vi "Main Engine Stream Process.vi"(8 "error in (no error)":errorcluster, 10 "Refs":T1, 11 "Process in":refnum<class "Process.lvclass">) -> (0 "error out":errorcluster)   [LabVIEW 2019, in "CAN Streaming Support Engine.lvlib"]
uses:
  CAN Streaming Support Engine.lvlib
  <vilib>/NI/NIVS Inline Async API/_VS Inline Async API/Process/Process.lvclass
  Types/Engine Stream API Refs.ctl
  <vilib>/xnet/xnet.llb/XNET Frame CAN.ctl
  <vilib>/xnet/xnet.llb/XNET Frame Type CAN.ctl
  Types/Engine Stream State.ctl
  <vilib>/NI/NIVS Inline Async API/_VS Inline Async API/Process/Process.lvclass/Process.ctl
  <vilib>/NI/NIVS Inline Async API/_VS Inline Async API/Error Handling Process/SubVIs/Error.ConvertArray.vi
  <vilib>/xnet/xnet.llb/XNET Read (Frame CAN).vi
  <vilib>/Utility/SystemLogging/Write to System Log.vi
  <vilib>/xnet/xnet.llb/XNET Create Session (Frame Input Stream).vi
  <vilib>/ErrorRing/Error Ring.xnode
  <resource>/objmgr/xnet.rc
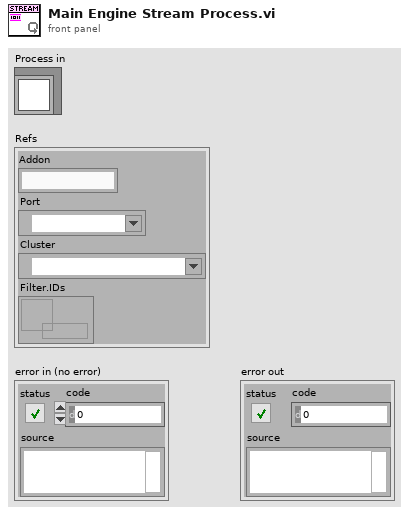
[diagram p1: front panel]
types:
  T1 = typedef "CAN Streaming Support Engine.lvlib/Engine Stream API Refs.ctl" = cluster{"Addon":string, "Port":refnum<k21>, "Cluster":refnum<k21>, "Filter.IDs":refnum<data-value>}
  T2 = typedef "CAN Streaming Support Engine.lvlib/Engine Stream State.ctl" = enum8{"Check for Connection", "Open XNET Session", "Publish", "Cleanup", "Exit"}
  T3 = typedef "XNET Frame CAN.ctl" = cluster{"timestamp":timestamp, "payload":u8[], "identifier":u32, "type":T4, "extended?":bool, "echo?":bool}
  T4 = typedef "XNET Frame Type CAN.ctl" = u8
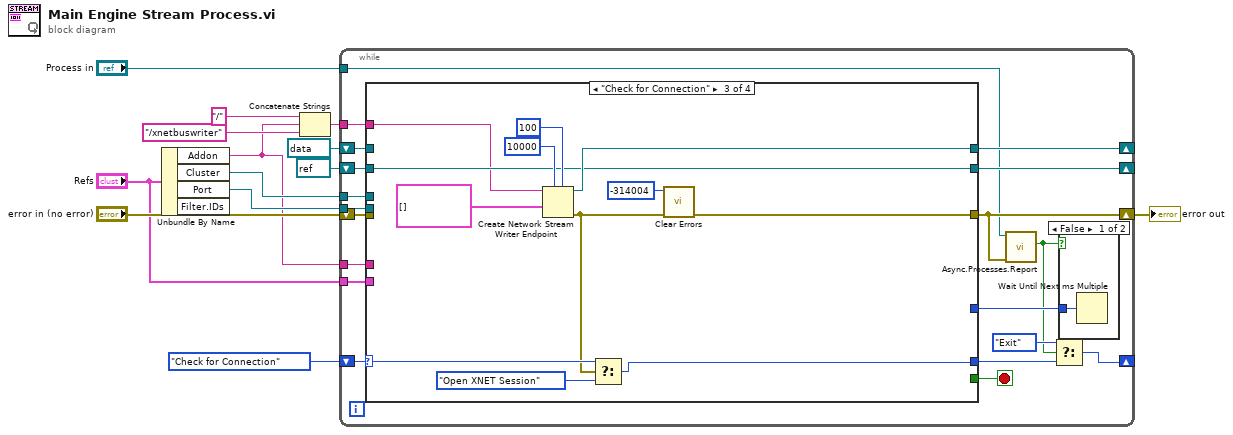
[diagram p0: block diagram]
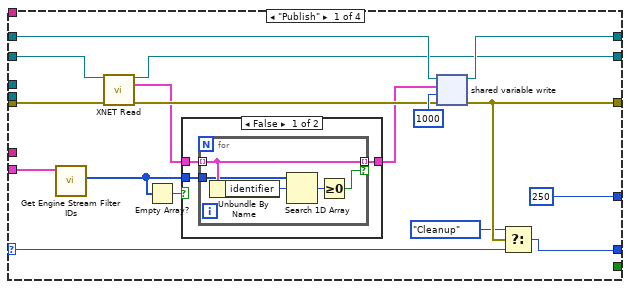
[diagram p2: hidden frame]
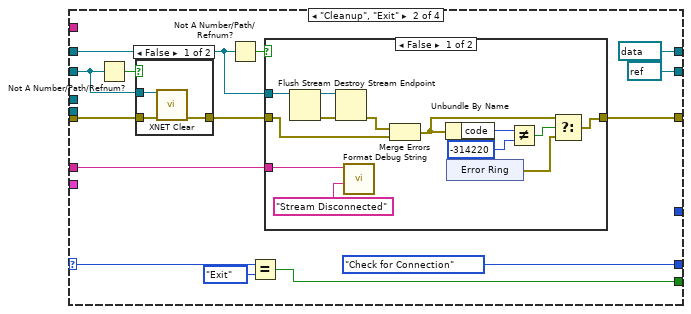
[diagram p4: hidden frame]
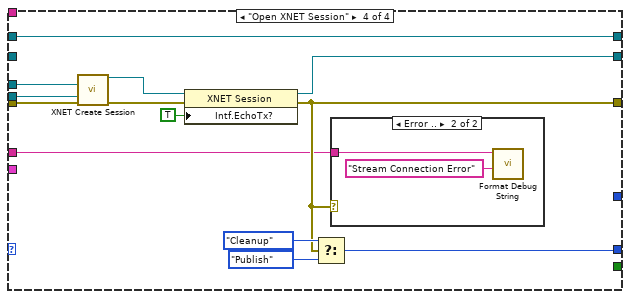
[diagram p7: hidden frame]
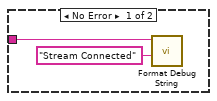
[diagram p8: hidden frame]
diagram:
  n1 = Unbundle By Name("Refs") -> ("Addon"=w1:string, "Cluster"=w13:refnum<k21>, "Port"=w12:refnum<k21>)  [unwired: 1 out]
  n2 = Concatenate Strings("/" ("string"), w1, "/xnetbuswriter" ("reader url")) -> (w8:string)
  n3 = while {
    shift-right: [w18] -> _
    shift-left: Engine_Stream_State."Check for Connection" -> [w32]
    shift-right: [w31] -> _
    shift-left: refnum<k21> refnum ("reader url") -> [w30]
    shift-right: [w21] -> w6
    shift-left: "error in (no error)" -> [w29]
    tunnel: w12 -> [w27]
    shift-right: [w26] -> _
    shift-left: refnum<k21> refnum ("session out") -> [w25]
    tunnel: w8 -> [w23]
    tunnel: w13 -> [w22]
    tunnel: "Process in" -> [w17]
    tunnel: "Refs" -> [w15]
    tunnel: w1 -> [w14]
    stop <- w28 stop-if-true
    n4 = case shown="\"Check for Connection\"" w32 {
      selector: w32 -> [w45 w70 w100 _]
      tunnel: [w44 Engine_Stream_State."Check for Connection" w98 w106] -> w19
      tunnel: [w47 refnum<k21> refnum ("reader url") w97 w107] -> w31
      tunnel: w30 -> [w48 w67 _ w107]
      tunnel: [w46 w60 w93 w105] -> w21
      tunnel: w29 -> [w36 w62 _ w116]
      tunnel: [_ w68 _ _] -> w28
      tunnel: w27 -> [_ _ _ w115]
      tunnel: [w39 refnum<k21> refnum ("session out") w96 w111] -> w26
      tunnel: w25 -> [w42 w64 w96 _]
      tunnel: [u32 250 ("millisecond multiple") _ _ _] -> w24
      tunnel: w23 -> [_ _ w95 _]
      tunnel: w22 -> [_ _ _ w112]
      tunnel: w15 -> [w34 _ _ _]
      tunnel: w14 -> [_ w59 _ w104]
      frame "Publish" {
        n5 = call "Get Engine Stream Filter IDs.vi"("Refs"=w34) -> ("IDs"=w33:u32[])  [unwired: 9 in, 1 out]
        n6 = call-poly <vilib>:"XNET Read.vi"("session in"=w42, "error in (no error)"=w36) -> ("session out"=w39:refnum<k21>, "data"=w35:T3[], "error out"=w41:errorcluster)  [unwired: 11 out]
        n7 = Empty Array?(array=w33) -> (empty?=w37:bool)
        n8 = case shown="False" w37 {
          tunnel: w35 -> [w52 w58]
          tunnel: [w51 w58] -> w38
          tunnel: w33 -> [w50 _]
          frame False {
            n9 = for {
              tunnel: w52 -> [w56] mode=indexing
              tunnel: w50 -> [w55]
              tunnel: [w56] -> w51 mode=indexing if=w53
              n10 = Unbundle By Name(w56) -> ("identifier"=w57:u32)
              n11 = Search 1D Array(1D array=w55, element=w57) -> (index of element=w54:i32)  [unwired: 1 in]
              n12 = Greater Or Equal To 0?(x=w54) -> (x >= 0?=w53:bool)
            }
          }
          frame True {
          }
        }
        n13 = shared-variable-write(w48, w41, w38, 1000 ("timeout ms")) -> (w47:refnum<k21>, w46:errorcluster)  [unwired: 1 out]
        n14 = Select(t=Engine_Stream_State."Cleanup", s=w46, f=w45) -> (s? t:f=w44:T2)
      }
      frame "Cleanup", "Exit" {
        n15 = Not A Number/Path/Refnum?(number/path/refnum=w64) -> (NaN/Path/Refnum?=w63:bool)
        n16 = case shown="False" w63 {
          tunnel: w62 -> [w75 w76]
          tunnel: [w74 w76] -> w61
          tunnel: w64 -> [w73 _]
          frame False {
            n17 = call <vilib>:"XNET Clear.vi"("session in"=w73, "error in (no error)"=w75) -> ("error out"=w74:errorcluster)  [unwired: 13 in]
          }
          frame True {
          }
        }
        n18 = Not A Number/Path/Refnum?(number/path/refnum=w67) -> (NaN/Path/Refnum?=w66:bool)
        n19 = Equal?(x=w70, y=Engine_Stream_State."Exit") -> (x = y?=w68:bool)
        n20 = case shown="False" w66 {
          tunnel: w61 -> [w81 w91]
          tunnel: [w83 w91] -> w60
          tunnel: w67 -> [w82 _]
          tunnel: w59 -> [w79 _]
          frame False {
            n21 = Flush Stream(11:w82) -> (0:w88:errorcluster, 3:w89:refnum<k21>)  [unwired: 3 in, 1 out]
            n22 = Destroy Stream Endpoint(8:w88, 11:w89) -> (0:w78:errorcluster)
            n23 = call "Format Debug String.vi"("State"="Stream Disconnected", "Name"=w79) -> ()  [unwired: 9 in, 1 out]
            n24 = Merge Errors(w78, w81) -> (w77:errorcluster)
            n25 = Unbundle By Name(w77) -> ("code"=w87:i32)
            n26 = xnode "Error Ring"() -> ("error out"=w84:errorcluster)
            n27 = Not Equal?(x=w87, y=-314220) -> (x != y?=w85:bool)
            n28 = Select(t=w77, s=w85, f=w84) -> (s? t:f=w83:errorcluster)
          }
          frame True {
          }
        }
      }
      frame "Check for Connection" {
        n29 = Create Network Stream Writer Endpoint(5:100 ("timeout in ms (-1)"), 7:10000 ("writer buffer size"), 9:T3[] [] ("data"), 11:w95) -> (0:w94:errorcluster, 3:w97:refnum<k21>)  [unwired: 3 in]
        n30 = Select(t=w100, s=w94, f=Engine_Stream_State."Open XNET Session") -> (s? t:f=w98:T2)
        n31 = call <vilib>:"Clear Errors.vi"("error in (no error)"=w94, "specific error code to clear (0: all)"=-314004) -> ("error out"=w93:errorcluster)  [unwired: 4 in, 1 out]
      }
      frame "Open XNET Session" {
        n32 = call-poly <vilib>:"XNET Create Session.vi"("cluster (:memory:)"=w112, "interface"=w115, "error in (no error)"=w116) -> ("session out"=w109:refnum<k21>, "error out"=w110:errorcluster)  [unwired: 11 out]
        n33 = property class="XNET Session"(reference=w109, error in=w110, "Intf.EchoTx?"=TRUE ("Interface:Echo Transmit?")) -> (reference out=w111:refnum<k21>, error out=w105:errorcluster)
        n34 = Select(t=Engine_Stream_State."Cleanup", s=w105, f=Engine_Stream_State."Publish") -> (s? t:f=w106:T2)
        n35 = case shown="Error .." w105 {
          tunnel: w104 -> [w118 w119]
          frame No Error {
            n36 = call "Format Debug String.vi"("State"="Stream Connected", "Name"=w118) -> ()  [unwired: 9 in, 1 out]
          }
          frame Error {
            n37 = call "Format Debug String.vi"("State"="Stream Connection Error", "Name"=w119) -> ()  [unwired: 9 in, 1 out]
          }
        }
      }
    }
    n38 = call <vilib>:"Async.Processes.Report.vi"("Error"=w21, "Process in"=w17) -> ("Stop"=w16:bool)  [unwired: 8 in, 1 out]
    n39 = Select(t=Engine_Stream_State."Exit" ("y"), s=w16, f=w19) -> (s? t:f=w18:T2)
    n40 = case shown="False" w16 {
      tunnel: w24 -> [w121 _]
      frame False {
        n41 = Wait Until Next ms Multiple(millisecond multiple=w121) -> ()  [unwired: 1 out]
      }
      frame True {
      }
    }
  }
  "error out" <- w6
